vi "Process.vi"(8 "error in (no error)":errorcluster, 10 "Pound in":refnum<class "Pound.lvclass">, 11 "Qbus in":refnum<class "Qbus.lvclass">) -> (0 "error out":errorcluster)   [LabVIEW 2017, in "IrDataEventCreator.lvlib"]
uses:
  <vilib>/addons/InsightCM/Devices/Shared/Ir/IrDataEventCreator/IrDataEventCreator.lvlib
  <vilib>/addons/Qbus/Qbus.lvclass
  <vilib>/NI/Software Watchdog/Pound/Pound.lvclass
  <vilib>/addons/InsightCM/Devices/Shared/Ir/IrDataEventCreator/controls/config.ctl
  <vilib>/addons/TraceLogger/TraceLogger.lvlib
  <vilib>/NI/Software Watchdog/Watchdog/Watchdog.lvclass
  <vilib>/addons/InsightCM/Devices/Shared/Common/DataFlow/DataFlow.lvlib
  <vilib>/addons/InsightCM/Utilities/GlobalConfiguration/GlobalConfiguration.lvlib
  <vilib>/addons/InsightCM/Devices/Shared/Common/DataEventCreator/DataEventCreator.lvlib
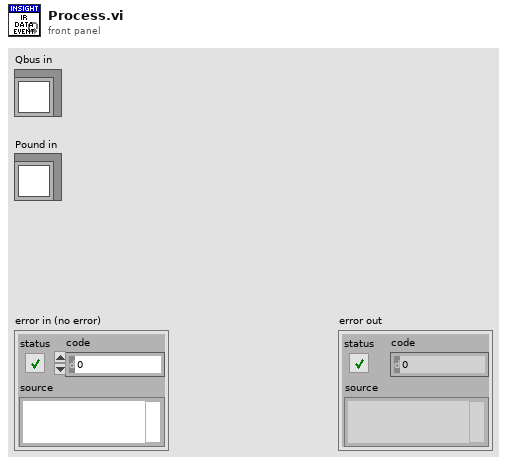
[diagram p1: front panel]
types:
  T1 = typedef "IrDataEventCreator.lvlib/config.ctl" = cluster{"Registry":variant, "CameraId Map":variant, "Device Name":string}
  T2 = typedef "IrDataEventCreator.lvlib/RegisterImageRoutedMessage.ctl" = cluster{"Name":string, "Image Registry":T3}
  T3 = typedef "IrDataEventCreator.lvlib/Registry_Image.ctl" = cluster{"Properties":T4[]}
  T4 = typedef "KeyValuePair.ctl" = cluster{"Key":string, "Value":string}
  T5 = typedef "DataEventCreator.lvlib/RegisterTrendPoints.ctl" = cluster{"DataGroup":string, "Trends":T6[]}
  T6 = typedef "DataEventCreator.lvlib/Registry_Trend.ctl" = cluster{"TrendPointId":string, "DataSetName":string, "HighRate":bool, "Always Send":bool}
  T7 = typedef "DataFlow.lvlib/Data.ctl" = cluster{"DataGroup":string, "Waveforms":T8, "Map":T9, "Type":T10}
  T8 = typedef "wfmSGL_DVR.ctl" = refnum<data-value>
  T9 = typedef "PointValueMap.lvlib/PointMap.ctl" = refnum<data-value>
  T10 = typedef "DataFlow.lvlib/Type.ctl" = enum16{"High Rate", "Low Rate", "Burst Mode"}
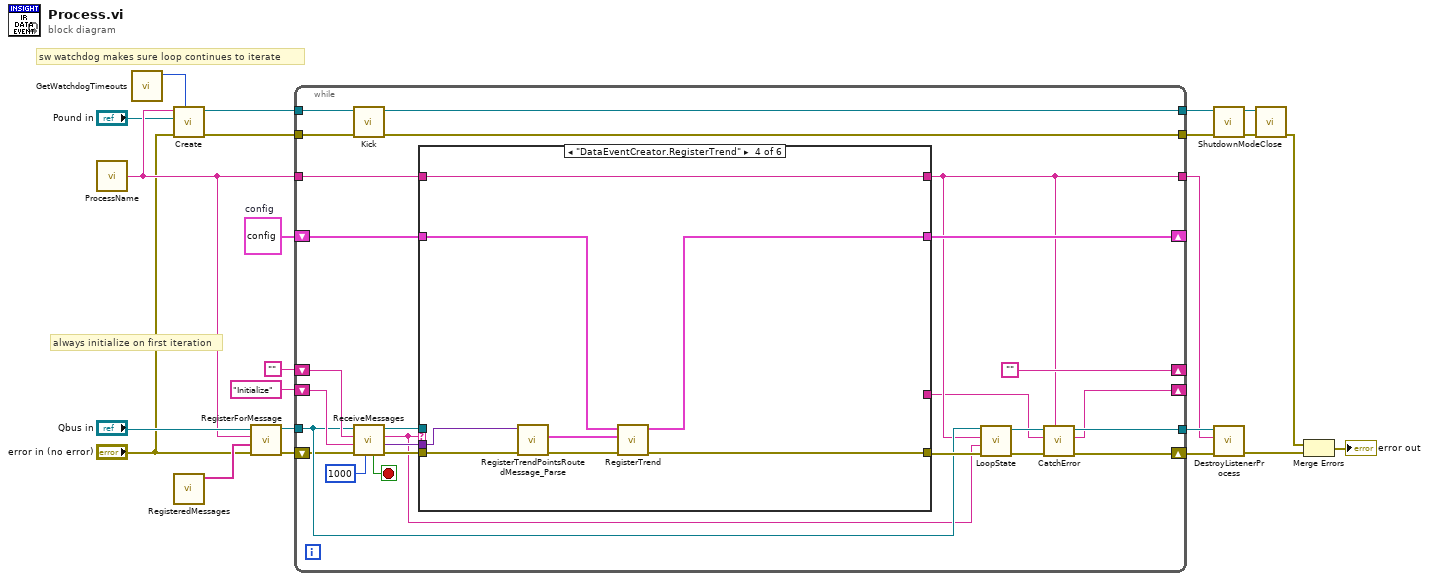
[diagram p0: block diagram]
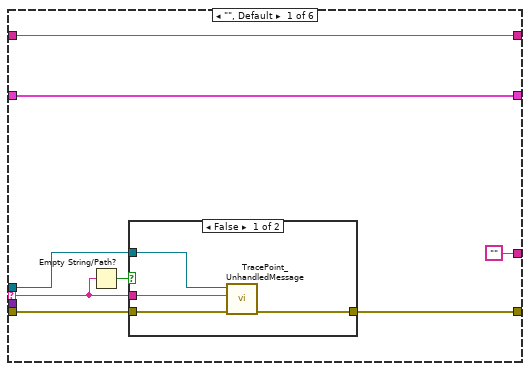
[diagram p2: hidden frame]
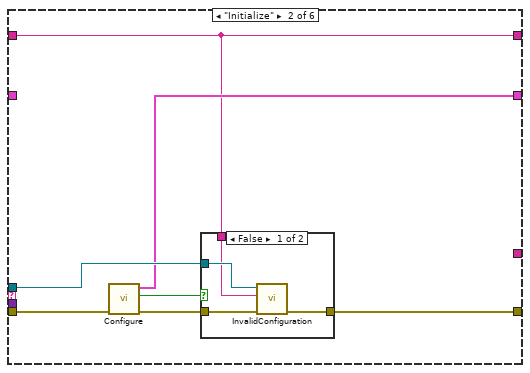
[diagram p4: hidden frame]
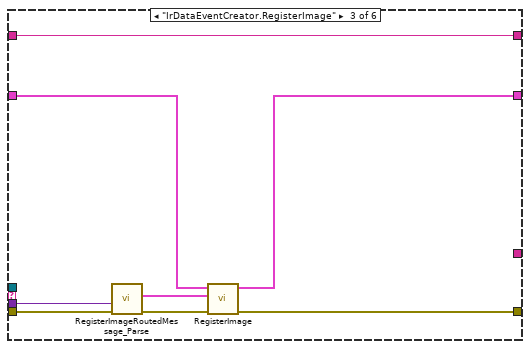
[diagram p6: hidden frame]
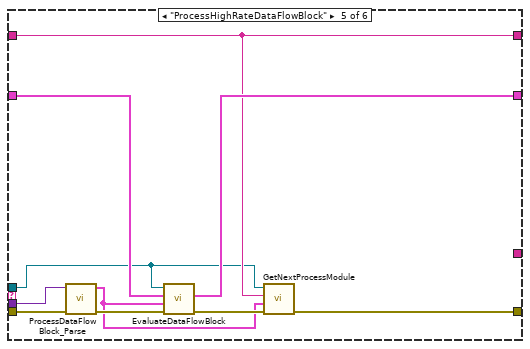
[diagram p7: hidden frame]
diagram:
  w15 = T1 {"Registry"=variant, "CameraId Map"=variant, "Device Name"=""}  # config
  # "always initialize on first iteration"
  # "sw watchdog makes sure loop continues to iterate"
  n1 = call <vilib>:"ProcessName.vi"() -> ("process name"=w13:string)  [unwired: 5 in]
  n2 = call <vilib>:"GetWatchdogTimeouts.vi"() -> ("software timeout"=w1:u32)  [unwired: 10 in, 1 out]
  n3 = call <vilib>:"Create.vi"("Execution Timeout (ms)"=w1, "error in (no error)"="error in (no error)", "Pound"="Pound in", "Name"=w13) -> ("error out"=w7:errorcluster, "Watchdog"=w12:refnum<data-value>)  [unwired: 6 in]
  n4 = call <vilib>:"RegisteredMessages.vi"() -> ("registered messages"=w14:string[])  [unwired: 11 in]
  n5 = call <vilib>:"RegisterForMessage.vi"("error in (no error)"="error in (no error)", "message names"=w14, "process name"=w13, "Qbus in"="Qbus in") -> ("error in (no error)"=w22:errorcluster, "Qbus out"=w21:refnum<class "Qbus.lvclass">)  [unwired: 6 in]
  n6 = while {
    shift-right: [""] -> _
    shift-left: "" -> [w48]
    tunnel: w21 -> [w36]
    tunnel: w13 -> [w26]
    tunnel: [w39] -> w19
    tunnel: [w25] -> w18
    shift-right: [w38] -> _
    shift-left: "Initialize" -> [w43]
    shift-right: [w41] -> _
    shift-left: w15 -> [w42]
    tunnel: w12 -> [w35]
    tunnel: [w34] -> w9
    tunnel: w7 -> [w33]
    tunnel: [w31] -> w6
    shift-right: [w40] -> w20
    shift-left: w22 -> [w32]
    stop <- w49 stop-if-true
    n7 = call <vilib>:"Kick.vi"("error in (no error)"=w33, "Watchdog"=w35) -> ("error out"=w31:errorcluster, "Watchdog"=w34:refnum<data-value>)  [unwired: 8 in]
    n8 = call <vilib>:"ReceiveMessages.vi"("Timeout(1000)"=1000 ("milliseconds to wait"), "error in (no error)"=w32, "priority action"=w43, "default action"=w48, "Qbus in"=w36) -> ("error out"=w47:errorcluster, "message value"=w44:variant, "action"=w30:string, "Qbus out"=w45:refnum<class "Qbus.lvclass">, "exit"=w49:bool)  [unwired: 2 in]
    n9 = case shown="\"DataEventCreator.RegisterTrend\"" w30 {
      selector: w30 -> [w53 _ _ _ _ _]
      tunnel: w47 -> [w55 w69 w80 w86 w99 w103]
      tunnel: w45 -> [w51 w67 _ _ w92 _]
      tunnel: [w54 w64 w75 w87 w94 w103] -> w37
      tunnel: w44 -> [_ _ w81 w85 w100 _]
      tunnel: w42 -> [w57 _ w77 w89 w97 w102]
      tunnel: [w57 w65 w76 w88 w96 w102] -> w41
      tunnel: [w56 w63 w82 w90 w93 w101] -> w25
      tunnel: w26 -> [w56 w63 w82 w90 w93 w101]
      tunnel: ["" _ _ _ _ _] -> w24
      frame "", Default {
        n10 = Empty String/Path?(string/path=w53) -> (empty?=w52:bool)
        n11 = case shown="False" w52 {
          tunnel: [w59 w62] -> w54
          tunnel: w55 -> [w60 w62]
          tunnel: w53 -> [w61 _]
          tunnel: w51 -> [w58 _]
          frame False {
            n12 = call <vilib>:"TracePoint_UnhandledMessage.vi"("error in (no error)"=w60, "message"=w61, "Qbus in"=w58) -> ("error out"=w59:errorcluster)  [unwired: 8 in]
          }
          frame True {
          }
        }
      }
      frame "Initialize" {
        n13 = call <vilib>:"Configure.vi"("error in (no error)"=w69) -> ("error out"=w68:errorcluster, "valid config"=w66:bool, "config"=w65:T1)  [unwired: 8 in]
        n14 = case shown="False" w66 {
          tunnel: w68 -> [w73 w74]
          tunnel: w67 -> [w72 _]
          tunnel: [w71 w74] -> w64
          tunnel: w63 -> [w70 _]
          frame False {
            n15 = call <vilib>:"InvalidConfiguration.vi"("error in (no error)"=w73, "description"=w70, "Qbus in"=w72) -> ("error out"=w71:errorcluster)  [unwired: 7 in, 1 out]
          }
          frame True {
          }
        }
      }
      frame "IrDataEventCreator.RegisterImage" {
        n16 = call <vilib>:"RegisterImageRoutedMessage_Parse.vi"("error in (no error)"=w80, "message"=w81) -> ("error out"=w79:errorcluster, "RegisterImageRoutedMessage data"=w78:T2)  [unwired: 8 in]
        n17 = call <vilib>:"RegisterImage.vi"("error in"=w79, "RegisterImageRoutedMessage data"=w78, "config"=w77) -> ("error out"=w75:errorcluster, "config"=w76:T1)  [unwired: 7 in]
      }
      frame "DataEventCreator.RegisterTrend" {
        n18 = call <vilib>:"RegisterTrendPointsRoutedMessage_Parse.vi"("error in (no error)"=w86, "message"=w85) -> ("error out"=w84:errorcluster, "RegisterTrend"=w83:T5)  [unwired: 8 in]
        n19 = call <vilib>:"RegisterTrend.vi"("error in"=w84, "RegisterTrend"=w83, "config"=w89) -> ("error out"=w87:errorcluster, "config"=w88:T1)  [unwired: 7 in]
      }
      frame "ProcessHighRateDataFlowBlock" {
        n20 = call <vilib>:"ProcessDataFlowBlock_Parse.vi"("error in (no error)"=w99, "body"=w100) -> ("error out"=w98:errorcluster, "data"=w91:T7)  [unwired: 8 in]
        n21 = call <vilib>:"EvaluateDataFlowBlock.vi"("error in (no error)"=w98, "data"=w91, "config in"=w97, "Qbus"=w92) -> ("error out"=w95:errorcluster, "config out"=w96:T1)  [unwired: 6 in]
        n22 = call <vilib>:"GetNextProcessModule.vi"("error in (no error)"=w95, "data"=w91, "source"=w93, "Qbus in"=w92) -> ("error out"=w94:errorcluster)  [unwired: 6 in, 1 out]
      }
      frame "Exit" {
      }
    }
    n23 = call <vilib>:"LoopState.vi"("error in (no error)"=w37, "loop action"=w30, "process name"=w25, "Qbus in"=w36) -> ("error out"=w28:errorcluster, "Qbus out"=w27:refnum<class "Qbus.lvclass">)  [unwired: 6 in]
    n24 = call <vilib>:"CatchError.vi"("source"=w25, "error in (no error)"=w28, "next action in"=w24, "Qbus in"=w27) -> ("error out"=w40:errorcluster, "next action out"=w38:string, "Qbus out"=w39:refnum<class "Qbus.lvclass">)  [unwired: 5 in]
  }
  n25 = call <vilib>:"ShutdownMode.vi"("error in (no error)"=w6, "Watchdog"=w9) -> ("error out"=w8:errorcluster, "Watchdog"=w10:refnum<data-value>)  [unwired: 8 in]
  n26 = call <vilib>:"DestroyListenerProcess.vi"("error in (no error)"=w20, "process name"=w18, "Qbus in"=w19) -> ("error in (no error)"=w5:errorcluster)  [unwired: 7 in, 1 out]
  n27 = call <vilib>:"Close.vi"("error in (no error)"=w8, "Watchdog"=w10) -> ("error out"=w4:errorcluster)  [unwired: 9 in]
  n28 = Merge Errors(w4, w5) -> (→"error out":errorcluster)
